vi "Model - Get NStream.vi"(8 "error in (no error)":errorcluster, 11 "View Model":T1) -> (0 "error out":errorcluster, 1 "exist?":bool, 2 "Endpoint":refnum<k21>, 3 "View Model":T1, 4 "AvailNSElmnts":i32, 5 "RTDataElmnts":i32)   [LabVIEW 2017]
doc: "Get actual value of Network Stream Endpoint from DVR"
uses:
  Controls/View Model.ctl
  Controls/Shared Model.ctl
  Error Handler/Controls/Error Model.ctl
  Error Handler/Controls/Error Event.ctl
  Error Handler/Controls/Error Type.ctl
  Controller/Controls/Controller Model.ctl
  Controller/Controls/Controller Event.ctl
  Controller/Controls/Controller Command.ctl
  Controller/Controls/Controller Overhead.ctl
  Real-Time/RT Status.ctl
  Real-Time/RT Loop Status.ctl
  Controller/Controls/Controller NStream.ctl
  Controller/Controls/Controller DAQ Data.ctl
  TDMS Logger/Controls/TDMS Model.ctl
  TDMS Logger/Controls/TDMS Event.ctl
  TDMS Logger/Controls/TDMS Command.ctl
  TDMS Logger/Controls/TDMS Overhead.ctl
  TDMS Logger/Controls/TDMS ChanProperties.ctl
  TDMS Logger/Controls/TDMS DAQ Data.ctl
  <resource>/objmgr/ni.dex.rc
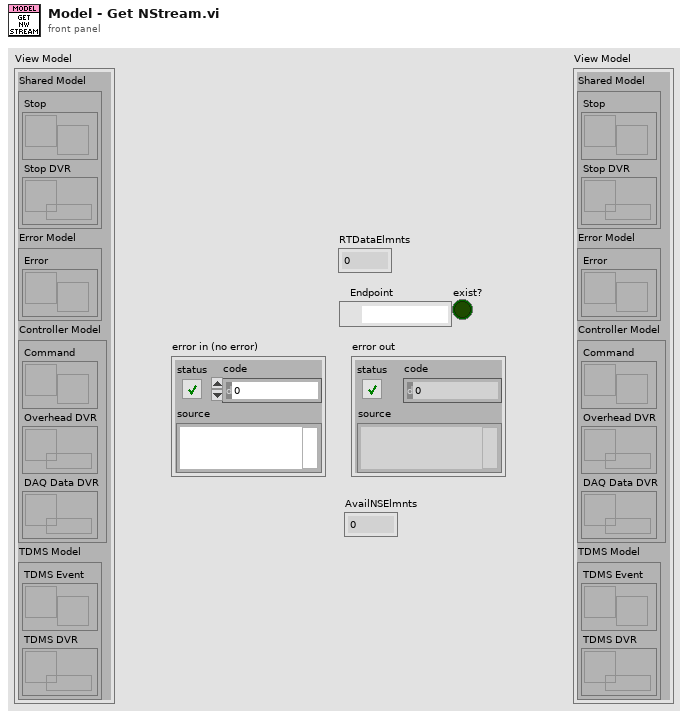
[diagram p1: front panel]
types:
  T1 = typedef "View Model.ctl" = cluster{"Shared Model":T2, "Error Model":T3, "Controller Model":T4, "TDMS Model":T5}
  T2 = typedef "Shared Model.ctl" = cluster{"Stop":refnum<user-event>, "Stop DVR":refnum<data-value>}
  T3 = typedef "Error Model.ctl" = cluster{"Error":refnum<user-event>}
  T4 = typedef "Controller Model.ctl" = cluster{"Command":refnum<user-event>, "Overhead DVR":refnum<data-value>, "DAQ Data DVR":refnum<data-value>}
  T5 = typedef "TDMS Model.ctl" = cluster{"TDMS Event":refnum<user-event>, "TDMS DVR":refnum<data-value>}
  T6 = typedef "Controller Overhead.ctl" = cluster{"Start":bool, "Numeric":dbl, "Blink CNTRLR1":bool, "Blink CNTRLR2":bool, "RT Status":T7, "RT data":dbl[][], "NStream":T9}
  T7 = typedef "RT Status.ctl" = cluster{"Status TCL1":T8, "Status TCL2":T8, "Status NPL":T8, "Connected?":bool}
  T8 = typedef "RT Loop Status.ctl" = cluster{"Duration, us":dbl, "Late Counter":i32, "Timeout, us":u32}
  T9 = typedef "Controller NStream.ctl" = cluster{"Endpoint":refnum<k21>, "exist?":bool, "# elements":i32}
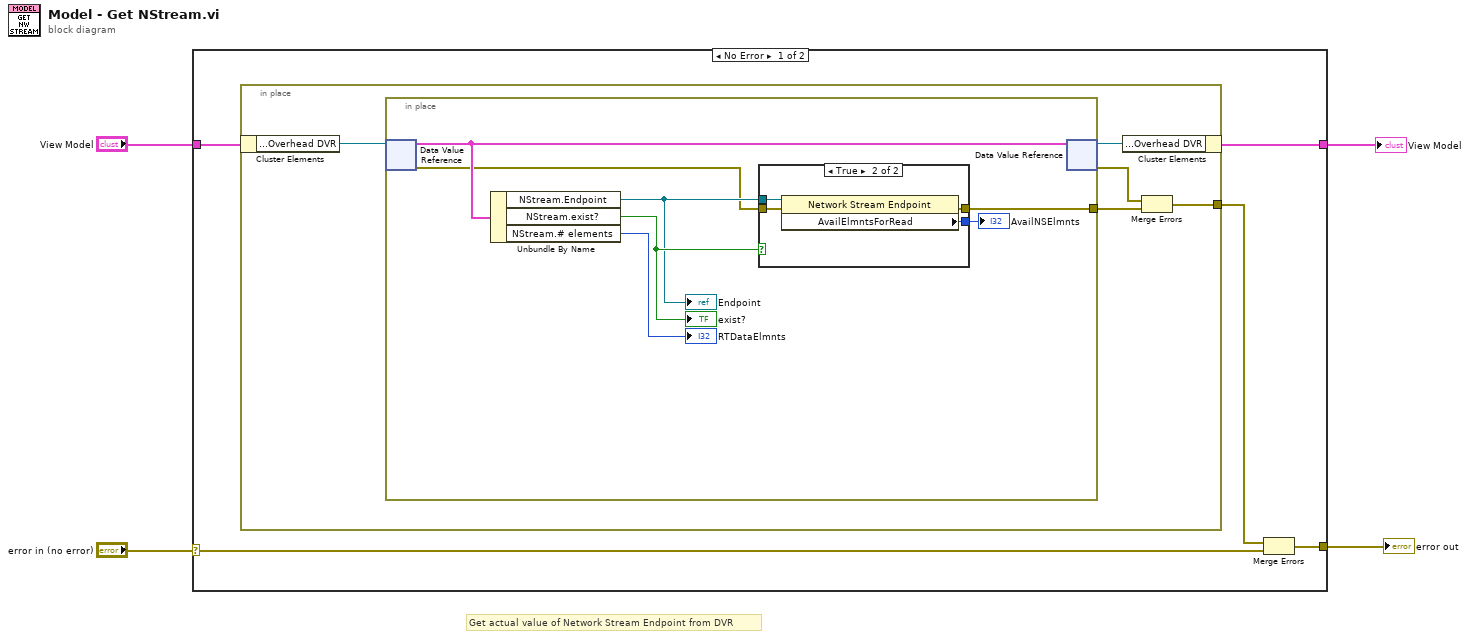
[diagram p0: block diagram]
diagram:
  # "Get actual value of Network Stream Endpoint from DVR"
  n1 = case shown="No Error" "error in (no error)" {
    selector: "error in (no error)" -> [w6 w27]
    tunnel: "View Model" -> [w9 w28]
    tunnel: [w8 w28] -> w2
    tunnel: [w5 w27] -> w1
    frame No Error {
      n2 = in-place {
        in-place-border: [w10] -> w7
        n3 = in-place-cluster #1(w9) -> ("Controller Model.Overhead DVR"=w14:refnum<data-value>)
        n4 = in-place {
          in-place-border: [w15] -> w12
          n5 = in-place-dvr #2(w14) -> (w21:T6, w17:errorcluster)
          n6 = Unbundle By Name(w21) -> ("NStream.Endpoint"=w18:refnum<k21>, "NStream.exist?"=w19:bool, "NStream.# elements"=→"RTDataElmnts":i32)
          "Endpoint" <- w18
          "exist?" <- w19
          n7 = case shown="True" w19 {
            tunnel: w17 -> [w22 w26]
            tunnel: w18 -> [_ w25]
            tunnel: [w22 w24] -> w15
            tunnel: [_ w23] -> w16
            frame False {
            }
            frame True {
              n8 = property class="Network Stream Endpoint"(reference=w25, error in=w26) -> (error out=w24:errorcluster, "AvailElmntsForRead"=w23:i32)  [unwired: 1 out]
            }
          }
          "AvailNSElmnts" <- w16
          n9 = in-place-dvr #2(w21) -> (w13:refnum<data-value>, w11:errorcluster)
        }
        n10 = in-place-cluster #1("Controller Model.Overhead DVR"=w13) -> (w8:T1)
        n11 = Merge Errors(w11, w12) -> (w10:errorcluster)
      }
      n12 = Merge Errors(w7, w6) -> (w5:errorcluster)
    }
    frame Error {
    }
  }
  "View Model" <- w2
  "error out" <- w1
